vi "generate_2_b.vi"() -> ()   [LabVIEW 2023]
uses:
  <vilib>/Utility/error.llb/DialogType.ctl
panel:
  in  "stop":bool
  out "error out 2":errorcluster
  in  "error in":errorcluster
  out "Data":i32
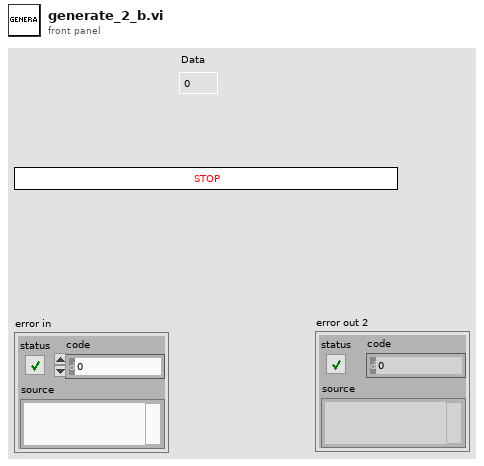
[diagram p1: front panel]
types:
  T1 = typedef "DialogType.ctl" = u16
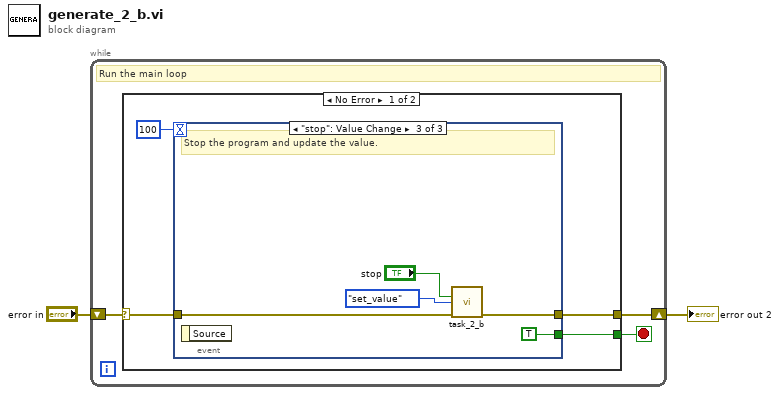
[diagram p0: block diagram]
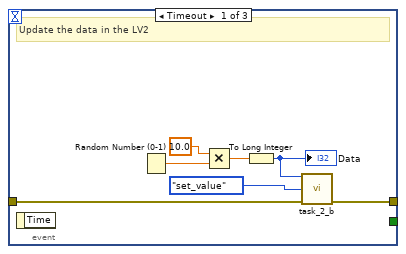
[diagram p2: hidden frame]
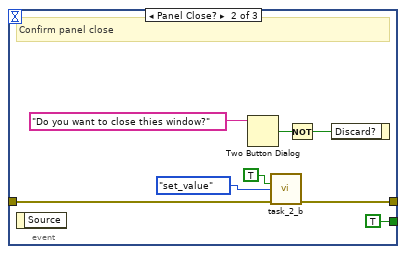
[diagram p3: hidden frame]
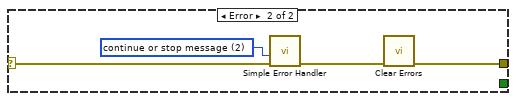
[diagram p4: hidden frame]
diagram:
  n1 = while {
    shift-right: [w4] -> w1
    shift-left: "error in" -> [w5]
    stop <- w3 stop-if-true
    # "Run the main loop"
    n2 = case shown="No Error" w5 {
      selector: w5 -> [w8 w33]
      tunnel: [w7 w31] -> w4
      tunnel: [w6 _] -> w3
      frame No Error {
        n3 = event shown="[2] \"stop\": Value Change" {
          selector: _ -> [_ _ _]
          dyn-events: _ -> [_ _ _]
          timeout: 100 -> [_ _ _]
          tunnel: [w10 w20 w28] -> w7
          tunnel: w8 -> [w11 w21 w29]
          tunnel: [_ TRUE TRUE] -> w6
          event Timeout {
            # "Update the data in the LV2"
            n4 = event-data() -> ()  [unwired: 1 in, 1 out]
            n5 = Random Number (0-1)() -> (number: 0 to 1=w16:dbl)
            n6 = Multiply(x=10.0, y=w16) -> (x*y=w14:dbl)
            n7 = To Long Integer(number=w14) -> (32bit integer=w13:i32)
            "Data" <- w13
            n8 = call "task_2_b.vi"("data"=w13, "Operation"=enum16{"get_value", "set_value", "Initialize"}."set_value", "error constant"=w11) -> ("error IO"=w10:errorcluster)  [unwired: 10 in, 2 out]
          }
          event Panel Close? {
            # "Confirm panel close"
            n9 = event-data() -> ()  [unwired: 1 in, 1 out]
            n10 = Two Button Dialog(message="Do you want to close thies window?") -> (T button?=w23:bool)  [unwired: 2 in]
            n11 = call "task_2_b.vi"("Stop"=TRUE, "Operation"=enum16{"get_value", "set_value", "Initialize"}."set_value", "error constant"=w21) -> ("error IO"=w20:errorcluster)  [unwired: 10 in, 2 out]
            n12 = Not(x=w23) -> (.not. x?=w22:bool)
            n13 = event-data("Discard?"=w22) -> ()  [unwired: 1 in, 1 out]
          }
          event "stop": Value Change {
            # "Stop the program and update the value."
            n14 = event-data() -> ()  [unwired: 1 in, 1 out]
            n15 = call "task_2_b.vi"("Stop"="stop", "Operation"=enum16{"get_value", "set_value", "Initialize"}."set_value", "error constant"=w29) -> ("error IO"=w28:errorcluster)  [unwired: 10 in, 2 out]
          }
        }
      }
      frame Error {
        w30 = T1 2 items=["no dialog", "OK message", "continue or stop message", "OK message + warnings", "continue/stop + warnings"] ("type of dialog (OK msg:1)")
        n16 = call <vilib>:"Simple Error Handler.vi"("type of dialog (OK msg:1)"=w30, "error in (no error)"=w33) -> ("error out"=w32:errorcluster)  [unwired: 3 in, 4 out]
        n17 = call <vilib>:"Clear Errors.vi"("error in (no error)"=w32) -> ("error out"=w31:errorcluster)  [unwired: 5 in, 1 out]
      }
    }
  }
  "error out 2" <- w1
